vi "String to Time.vi"(8 "error in (no error)":errorcluster, 10 "Include ms":bool=TRUE, 11 "String to Convert":string) -> (0 "error out":errorcluster, 3 "Time Value":timestamp)   [LabVIEW 2023, in "HAF.lvlib"]
doc: "Convert a String representation of a Timestamp to a Time, ignoring the date. The date will be set to 01/01/1904. The passed string must be in the format HH:MM:SS.fff otherwise an invalid converstion or other error will be raised. The time can include any passed milliseconds or be set to zero."
uses:
  HAF.lvlib
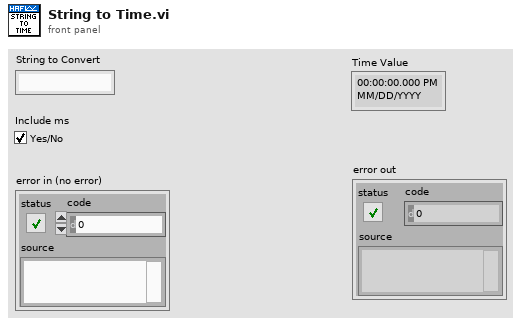
[diagram p1: front panel]
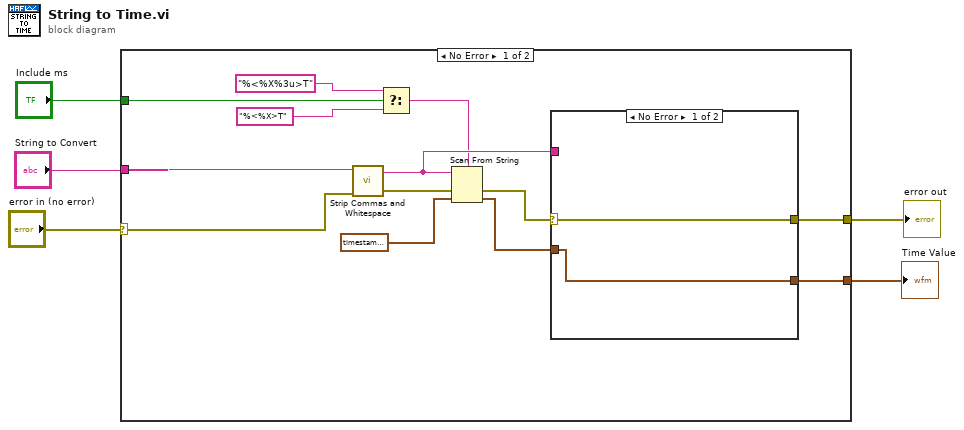
[diagram p0: block diagram]
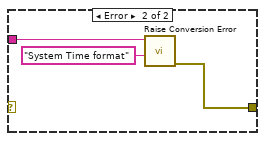
[diagram p2: hidden frame]
diagram:
  n1 = case shown="No Error" "error in (no error)" {
    selector: "error in (no error)" -> [w17 w24]
    tunnel: "String to Convert" -> [w18 _]
    tunnel: [w12 w24] -> w3
    tunnel: [w11 _] -> w2
    tunnel: "Include ms" -> [w9 _]
    frame No Error {
      n2 = call "Strip Commas and Whitespace.vi"("error in (no error)"=w17, "String to Strip"=w18) -> ("error out"=w16:errorcluster, "Clean String"=w10:string)  [unwired: 8 in]
      n3 = Select(t="%<%X%3u>T", s=w9, f="%<%X>T") -> (s? t:f=w6:string)
      n4 = Scan From String(format string=w6, input string=w10, error in=w16, default 1=timestamp(0 s since 1904-01-01)) -> (error out=w14:errorcluster, output 1=w13:timestamp)  [unwired: 1 in, 2 out]
      n5 = case shown="No Error" w14 {
        selector: w14 -> [w20 _]
        tunnel: w13 -> [w19 _]
        tunnel: [w20 w21] -> w12
        tunnel: [w19 _] -> w11
        tunnel: w10 -> [_ w23]
        frame No Error {
        }
        frame Error {
          n6 = call "Raise Conversion Error.vi"("Data Type Attempted"="System Time format", "String in Error"=w23) -> ("error out"=w21:errorcluster)  [unwired: 9 in]
        }
      }
    }
    frame Error {
    }
  }
  "Time Value" <- w2
  "error out" <- w3
